vi "Get COM Descriptor.vi"(7 "To ASCII? (True)":bool=TRUE, 8 "error in (no error)":errorcluster, 10 "Generate error if no COM port found? (False)":bool, 11 "COM name":string) -> (0 "error out":errorcluster, 2 "COM port Descriptor":string, 3 "COM port":T1)   [LabVIEW 2020, in "Get COM Descriptor.lvlib"]
doc: "Get COM port descriptor string. Option To ASCII? will try to remove utf8 symbols (replaces accents with basic alphabet).\n\nDetails: https://github.com/smaslan/get-com-descriptor"
uses:
  Get COM Descriptor.lvlib
  COM port.ctl
  <vilib>/Utility/error.llb/Error Cluster From Error Code.vi
  <vilib>/ErrorRing/Error Ring.xnode
  get_com_descriptor.dll
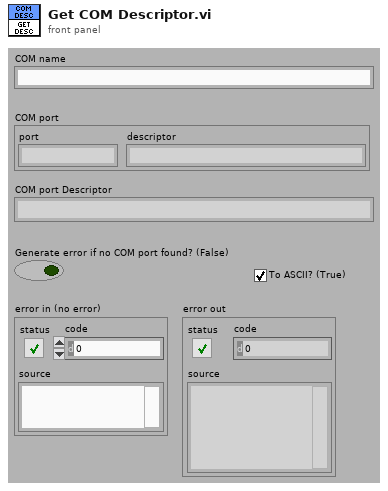
[diagram p1: front panel]
types:
  T1 = typedef "Get COM Descriptor.lvlib/COM port.ctl" = cluster{"port":string, "descriptor":string}
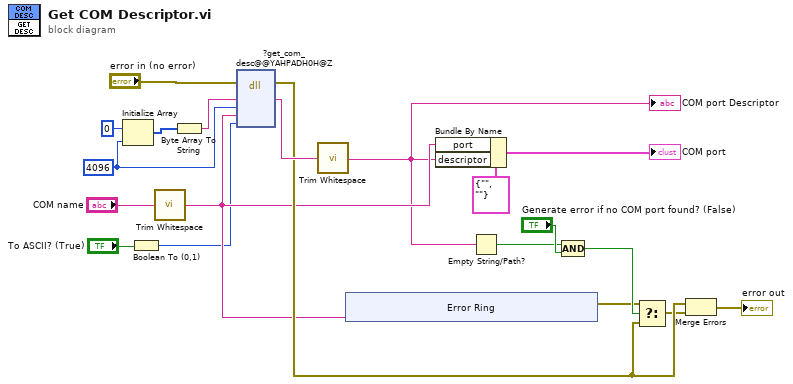
[diagram p0: block diagram]
diagram:
  w16 = 4096 ("dimension size")
  n1 = Initialize Array(u8 0 ("element"), w16) -> (w19:u8[])
  n2 = Boolean To (0,1)(Boolean="To ASCII? (True)") -> (0, 1=w1:i16)
  n3 = call <vilib>:"Trim Whitespace.vi"("string"="COM name") -> ("trimmed string"=w6:string)  [unwired: 1 in]
  n4 = Byte Array To String(unsigned byte array=w19) -> (string=w17:string)
  n5 = dll-call lib="F:/Z_bridge_v4/other/get_com_descriptor/get_com_descriptor.dll" fn="?get_com_desc@@YAHPADH0H@Z"(error in="error in (no error)", "buf"=w17, "size"=w16, "name"=w6, "to_ascii"=w1) -> (error out=w10:errorcluster, "buf"=w15:string)  [unwired: 6 in, 1 out]
  n6 = call <vilib>:"Trim Whitespace.vi"("string"=w15) -> ("trimmed string"=w4:string)  [unwired: 1 in]
  "COM port Descriptor" <- w4
  n7 = xnode "Error Ring"("parameter 0"=w6) -> ("error out"=w11:errorcluster)
  n8 = Bundle By Name(cluster=T1 {"port"="", "descriptor"=""} ("COM port"), "port"=w6, "descriptor"=w4) -> (→"COM port":T1)
  n9 = Empty String/Path?(string/path=w4) -> (empty?=w3:bool)
  n10 = Compound Arithmetic op=AND(w3, "Generate error if no COM port found? (False)") -> (w12:bool)
  n11 = Select(t=w11, s=w12, f=w10) -> (s? t:f=w9:errorcluster)
  n12 = Merge Errors(w10, w9) -> (→"error out":errorcluster)
